vi "Get Internal Tn.vi"(8 "error in":errorcluster, 11 "VISA resource name in":refnum<visa-resource-name>) -> (0 "error out":errorcluster, 1 "InternalTn (out)":u16, 3 "VISA resource name out":refnum<visa-resource-name>)   [LabVIEW 2018, in "JULABO DeviceDriver.lvlib"]
doc: "This VI returns the Resetting time <B>Tn</B> (Integral component) in case of internal temperature control."
uses:
  JULABO DeviceDriver.lvlib
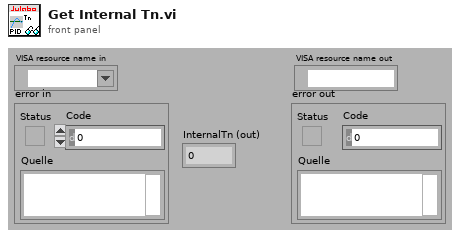
[diagram p1: front panel]
types:
  T1 = typedef "JULABO DeviceDriver.lvlib/InstrumentType.ctl" = enum8{"Default", "FC-Series", "HT30/HT60", "LC4"}
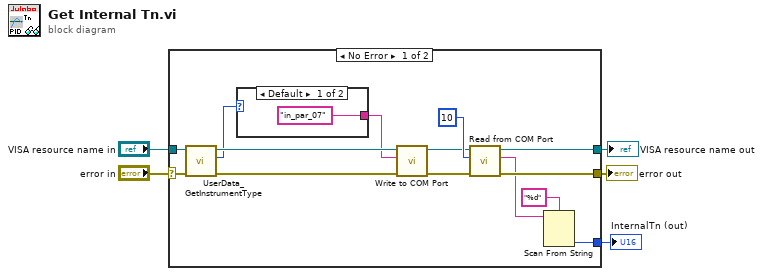
[diagram p0: block diagram]
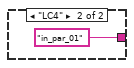
[diagram p2: hidden frame]
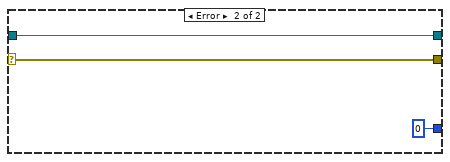
[diagram p3: hidden frame]
diagram:
  n1 = case shown="No Error" "error in" {
    selector: "error in" -> [w6 w23]
    tunnel: "VISA resource name in" -> [w7 w24]
    tunnel: [w19 w24] -> w4
    tunnel: [w18 w23] -> w3
    tunnel: [w14 0] -> w1
    frame No Error {
      n2 = call "UserData_GetInstrumentType.vi"("Fehler (Eingang)"=w6, "VISA resource name in"=w7) -> ("Fehler (Ausgang)"=w12:errorcluster, "InstrumentType"=w11:T1, "VISA resource name out"=w13:refnum<visa-resource-name>)  [unwired: 3 in]
      n3 = case shown="Default" w11 {
        tunnel: ["in_par_07" "in_par_01"] -> w10
        frame Default {
        }
        frame "LC4" {
        }
      }
      n4 = call "Write to COM Port.vi"("error in"=w12, "Command (input)"=w10, "VISA resource name in"=w13) -> ("error out"=w8:errorcluster, "VISA resource name out"=w9:refnum<visa-resource-name>)  [unwired: 7 in]
      n5 = call "Read from COM Port.vi"("error in"=w8, "Byte to Read (-1:All)"=u32 10 ("Anzahl der Byte"), "VISA resource name in"=w9) -> ("error out"=w18:errorcluster, "String (output)"=w15:string, "VISA resource name out"=w19:refnum<visa-resource-name>)  [unwired: 5 in, 1 out]
      n6 = Scan From String(format string="%d" ("Format-String"), input string=w15) -> (output 1=w14:i32)  [unwired: 3 in, 3 out]
    }
    frame Error {
    }
  }
  "VISA resource name out" <- w4
  "error out" <- w3
  "InternalTn (out)" <- w1
